vi "bmd101Parser_v1.vi"() -> ()   [LabVIEW 2016]
doc: "This example performs writes and reads on a serial port, as directed by the user. You can press the Write and Read buttons, and change the Read Count, while the example is running.\n\nThe parameters set for the serial port must match the parameters of the connected instrument or device. In this example, the Read Count parameter specifies the number of bytes that the serial port reads. If there were more bytes at the port than the specified number, those bytes would not be read. If there were less bytes at the port than the specified number, you would receive a timeout error.\n\nThis example expands upon the flow control options for XON and XOFF, allowing the user to choose those control characters. Also, the user can enable or disable a termination character. Some devices require a termination character in order to identify the end of command strings. Some devices send a termination character to signify the end of data to be read. This example shows how you can end the Read operation once a termination character is detected in the buffer and/or append a termination character at the end of the Write data."
uses:
  C:/Program Files/National Instruments/LabVIEW 2016/examples/Instrument IO/Serial/support/Serial - Settings.ctl
  <vilib>/Instr/_visa.llb/VISA Configure Serial Port (Instr).vi
panel:
  out "Waveform Chart":i16[](graph)
  out "return count":u32
  out "Response":string
  in  "Read Count":u32=800
  in  "Read":bool=TRUE
  in  "Stop":bool
  in  "Serial Settings":T1={"baud rate"=57600, "data bits"=8, "parity"=enum."None", "stop bits"=10, "flow control"=0} {"flow control" items=["None"=0, "XON/XOFF"=1, "RTS/CTS"=2, "DTR/DSR"=4]; "stop bits" items=["1.0"=10, "1.5"=15, "2.0"=20]; "data bits" min=5 max=8 step=1; "baud rate" items=["75"=75, "110"=110, "134"=134, "150"=150, "300"=300, "600"=600, "1200"=1200, "1800"=1800, "2400"=2400, "4800"=4800, "7200"=7200, "9600"=9600, "14400"=14400, "19200"=19200, "28800"=28800, "38400"=38400, "56000"=56000, "57600"=57600, "115200"=115200, "128000"=128000, "230400"=230400]}
  in  "VISA resource name":refnum<visa-resource-name>="bmd101"
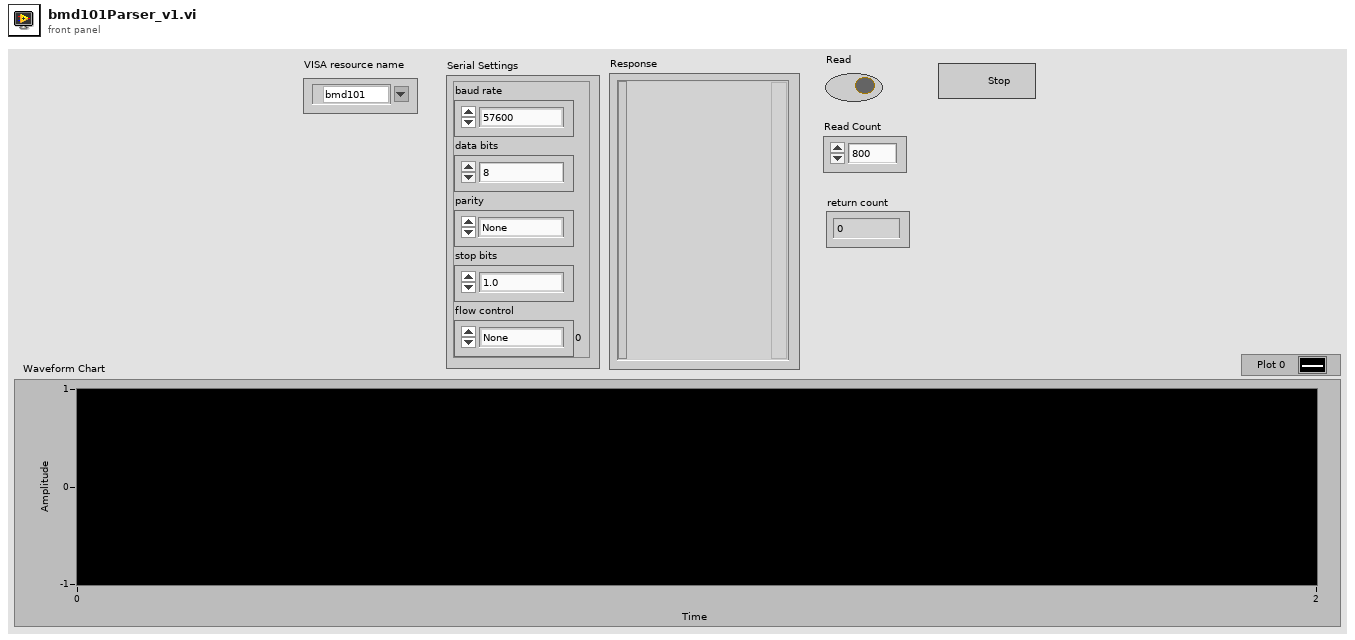
[diagram p1: front panel]
types:
  T1 = typedef "Serial - Settings.ctl" = cluster{"baud rate":u32, "data bits":u16, "parity":enum16{"None", "Odd", "Even", "Mark", "Space"}, "stop bits":u16, "flow control":u16}
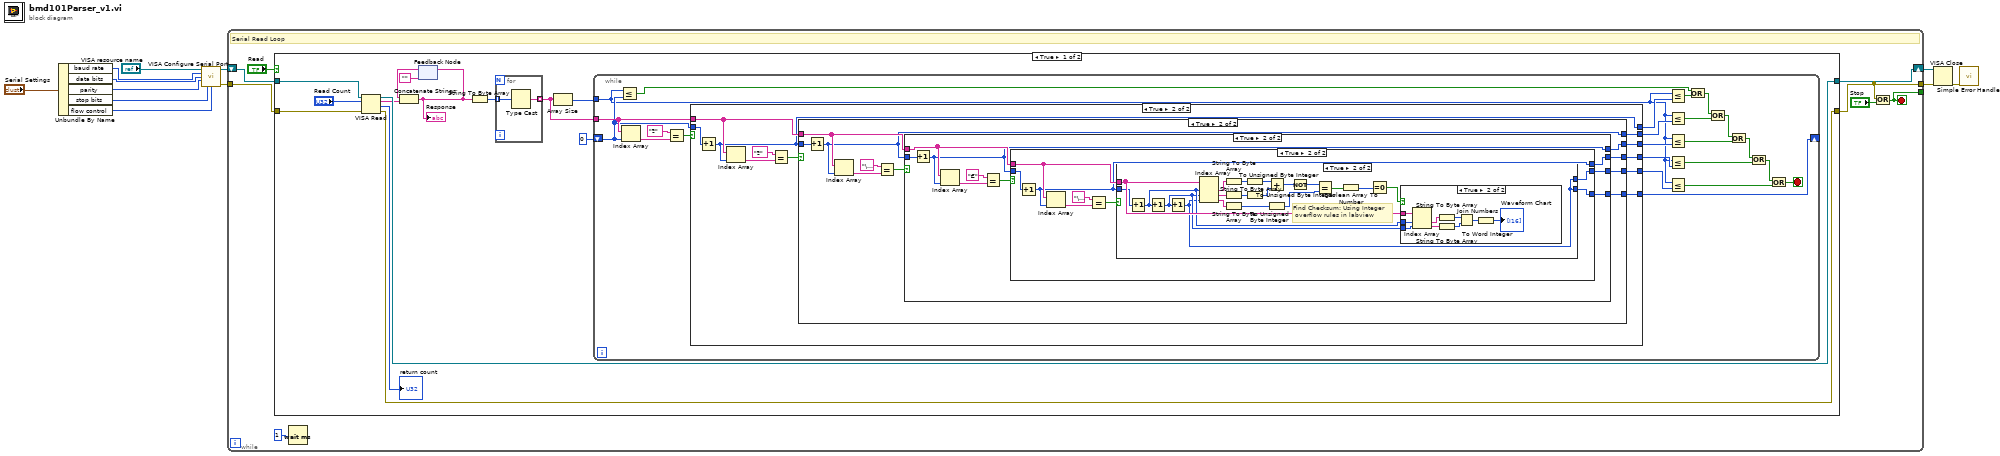
[diagram p0: block diagram]
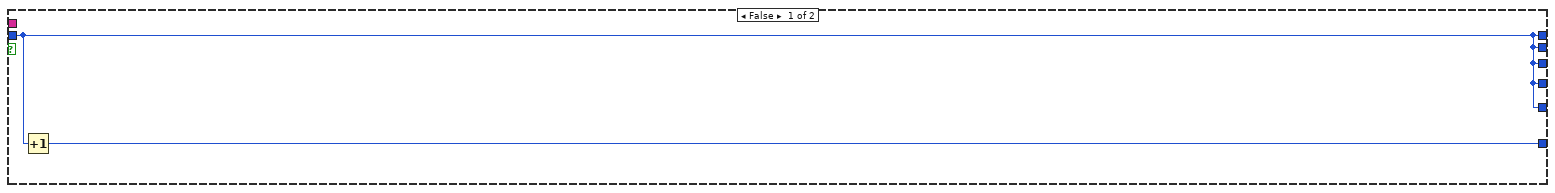
[diagram p2: hidden frame]
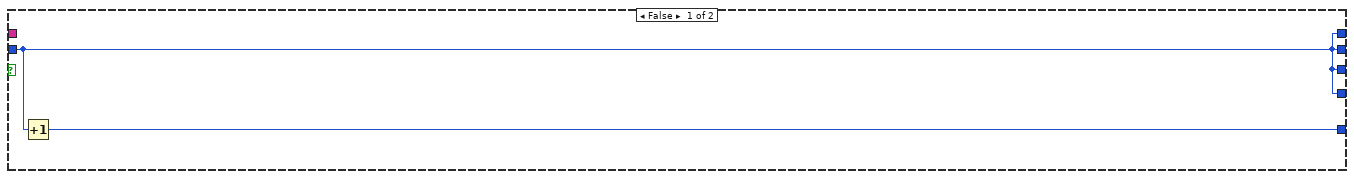
[diagram p3: hidden frame]
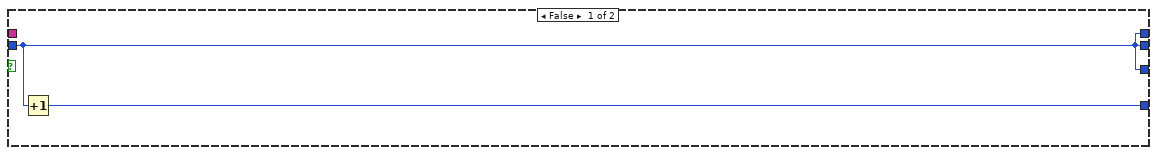
[diagram p4: hidden frame]
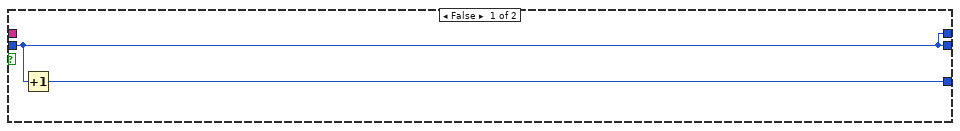
[diagram p5: hidden frame]
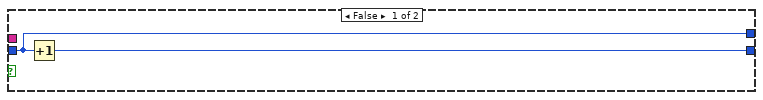
[diagram p6: hidden frame]
diagram:
  n1 = Unbundle By Name("Serial Settings") -> ("baud rate"=w11:u32, "data bits"=w10:u16, "parity"=w9:enum16{"None", "Odd", "Even", "Mark", "Space"}, "stop bits"=w8:u16, "flow control"=w7:u16)
  n2 = call-poly "VISA Configure Serial Port"("VISA resource name"="VISA resource name", "baud rate (9600)"=w11, "data bits (8)"=w10, "parity (0:none)"=w9, "stop bits (10: 1 bit)"=w8, "flow control (0:none)"=w7) -> ("VISA resource name out"=w3:refnum<visa-resource-name>, "error out"=w2:errorcluster)  [unwired: 4 in, 4 out]
  n3 = while {
    shift-right: [w20] -> w4
    shift-left: w3 -> [w15]
    tunnel: w2 -> [w14]
    tunnel: [w17] -> w5
    tunnel: [w13] -> _
    stop <- w13 stop-if-true
    # "Serial Read Loop"
    n4 = case shown="True" "Read" {
      tunnel: [w32 w137] -> w20
      tunnel: w15 -> [w34 w137]
      tunnel: [w30 w136] -> w17
      tunnel: w14 -> [w33 w136]
      frame True {
        n5 = VISA Read(VISA resource name=w34, byte count="Read Count", error in (no error)=w33) -> (VISA resource name out=w32:refnum<visa-resource-name>, read buffer=w29:string, return count=→"return count":u32, error out=w30:errorcluster)
        n6 = feedback #1("") -> (w28:string)
        n7 = Concatenate Strings(w28, w29) -> (w25:string)
        "Response" <- w25
        n8 = feedback-in #1(w25) -> ()
        n9 = String To Byte Array(string=w25) -> (unsigned byte array=w26:u8[])
        n10 = for {
          tunnel: w26 -> [w135] mode=indexing
          tunnel: [w134] -> w23 mode=indexing
          n11 = Type Cast(x=w135) -> (*(type *) &x=w134:string)  [unwired: 1 in]
        }
        n12 = Array Size(array=w23) -> (size(s)=w21:i32)
        n13 = while {
          tunnel: w23 -> [w53]
          shift-right: [w57] -> _
          shift-left: 0 -> [w52]
          tunnel: w21 -> [w38]
          stop <- w35 stop-if-true
          n14 = Less Or Equal?(x=w38, y=w52) -> (x <= y?=w50:bool)
          n15 = Index Array(array=w53, index=w52) -> (element=w56:string)
          n16 = Equal?(x="ª", y=w56) -> (x = y?=w54:bool)
          n17 = case shown="True" w54 {
            tunnel: w52 -> [w58 w68]
            tunnel: [w59 w66] -> w57
            tunnel: w53 -> [_ w65]
            tunnel: [w58 w64] -> w51
            tunnel: [w58 w63] -> w48
            tunnel: [w58 w62] -> w45
            tunnel: [w58 w61] -> w42
            tunnel: [w58 w60] -> w39
            frame False {
              n18 = Increment(x=w58) -> (x+1=w59:i32)
            }
            frame True {
              n19 = Increment(x=w68) -> (x+1=w64:i32)
              n20 = Index Array(array=w65, index=w64) -> (element=w70:string)
              n21 = Equal?(x="ª", y=w70) -> (x = y?=w67:bool)
              n22 = case shown="True" w67 {
                tunnel: w64 -> [w71 w82]
                tunnel: [w72 w78] -> w66
                tunnel: w65 -> [_ w77]
                tunnel: [w71 w76] -> w63
                tunnel: [w71 w75] -> w62
                tunnel: [w71 w74] -> w61
                tunnel: [w71 w73] -> w60
                frame False {
                  n23 = Increment(x=w71) -> (x+1=w72:i32)
                }
                frame True {
                  n24 = Increment(x=w82) -> (x+1=w76:i32)
                  n25 = Index Array(array=w77, index=w76) -> (element=w80:string)
                  n26 = Equal?(x="\u0004", y=w80) -> (x = y?=w79:bool)
                  n27 = case shown="True" w79 {
                    tunnel: w76 -> [w83 w90]
                    tunnel: [w84 w89] -> w78
                    tunnel: w77 -> [_ w88]
                    tunnel: [w83 w87] -> w75
                    tunnel: [w83 w86] -> w74
                    tunnel: [w83 w85] -> w73
                    frame False {
                      n28 = Increment(x=w83) -> (x+1=w84:i32)
                    }
                    frame True {
                      n29 = Increment(x=w90) -> (x+1=w87:i32)
                      n30 = Index Array(array=w88, index=w87) -> (element=w91:string)
                      n31 = Equal?(x="€", y=w91) -> (x = y?=w92:bool)
                      n32 = case shown="True" w92 {
                        tunnel: w87 -> [w94 w100]
                        tunnel: [w95 w99] -> w89
                        tunnel: w88 -> [_ w98]
                        tunnel: [w94 w97] -> w86
                        tunnel: [w94 w96] -> w85
                        frame False {
                          n33 = Increment(x=w94) -> (x+1=w95:i32)
                        }
                        frame True {
                          n34 = Increment(x=w100) -> (x+1=w97:i32)
                          n35 = Index Array(array=w98, index=w97) -> (element=w101:string)
                          n36 = Equal?(x="\u0002", y=w101) -> (x = y?=w102:bool)
                          n37 = case shown="True" w102 {
                            tunnel: w97 -> [w104 w109]
                            tunnel: [w105 w106] -> w99
                            tunnel: w98 -> [_ w110]
                            tunnel: [w104 w106] -> w96
                            frame False {
                              n38 = Increment(x=w104) -> (x+1=w105:i32)
                            }
                            frame True {
                              # "Find Checksum: Using Integer\n overflow rules in labview"
                              n39 = Increment(x=w109) -> (x+1=w108:i32)
                              n40 = Increment(x=w108) -> (x+1=w107:i32)
                              n41 = Increment(x=w107) -> (x+1=w106:i32)
                              n42 = Index Array(array=w110, index #1=w108, index #2=w107, index #3=w106) -> (element #1=w124:string, element #2=w123:string, element #3=w117:string)
                              n43 = String To Byte Array(string=w124) -> (unsigned byte array=w122:u8[])
                              n44 = String To Byte Array(string=w123) -> (unsigned byte array=w121:u8[])
                              n45 = String To Byte Array(string=w117) -> (unsigned byte array=w116:u8[])
                              n46 = To Unsigned Byte Integer(number=w122) -> (unsigned 8bit integer=w120:u8[])
                              n47 = To Unsigned Byte Integer(number=w121) -> (unsigned 8bit integer=w119:u8[])
                              n48 = Add(x=w120, y=w119) -> (x+y=w118:u8[])
                              n49 = To Unsigned Byte Integer(number=w116) -> (unsigned 8bit integer=w114:u8[])
                              n50 = Not(x=w118) -> (.not. x?=w115:u8[])
                              n51 = Equal?(x=w115, y=w114) -> (x = y?=w113:bool[])
                              n52 = Boolean Array To Number(Boolean array=w113) -> (number=w112:u32)
                              n53 = Equal To 0?(x=w112) -> (x = 0?=w111:bool)
                              n54 = case shown="True" w111 {
                                tunnel: w110 -> [_ w133]
                                tunnel: w108 -> [_ w126]
                                tunnel: w107 -> [_ w125]
                                frame False {
                                }
                                frame True {
                                n55 = Index Array(array=w133, index #1=w126, index #2=w125) -> (element #1=w132:string, element #2=w131:string)
                                n56 = String To Byte Array(string=w132) -> (unsigned byte array=w130:u8[])
                                n57 = String To Byte Array(string=w131) -> (unsigned byte array=w129:u8[])
                                n58 = Join Numbers(hi=w130, lo=w129) -> ((hi.lo)=w128:u16[])
                                n59 = To Word Integer(number=w128) -> (16bit integer=→"Waveform Chart":i16[])
                                }
                              }
                            }
                          }
                        }
                      }
                    }
                  }
                }
              }
            }
          }
          n60 = Less Or Equal?(x=w38, y=w51) -> (x <= y?=w49:bool)
          n61 = Less Or Equal?(x=w38, y=w48) -> (x <= y?=w46:bool)
          n62 = Less Or Equal?(x=w38, y=w45) -> (x <= y?=w43:bool)
          n63 = Less Or Equal?(x=w38, y=w42) -> (x <= y?=w40:bool)
          n64 = Less Or Equal?(x=w38, y=w39) -> (x <= y?=w36:bool)
          n65 = Or(x=w50, y=w49) -> (x .or. y?=w47:bool)
          n66 = Or(x=w47, y=w46) -> (x .or. y?=w44:bool)
          n67 = Or(x=w44, y=w43) -> (x .or. y?=w41:bool)
          n68 = Or(x=w41, y=w40) -> (x .or. y?=w37:bool)
          n69 = Or(x=w37, y=w36) -> (x .or. y?=w35:bool)
        }
      }
      frame False {
      }
    }
    n70 = Wait (ms)(milliseconds to wait=u32 1) -> ()  [unwired: 1 out]
    n71 = Or(x=w17, y="Stop") -> (x .or. y?=w13:bool)
  }
  n72 = VISA Close(VISA resource name=w4, error in (no error)=w5) -> (error out=w1:errorcluster)
  n73 = call <vilib>:"Simple Error Handler.vi"("error in (no error)"=w1) -> ()  [unwired: 1 in, 8 out]
